vi "PIO.Read (U64).vi"(8 "error in (no error)":errorcluster, 10 "offset":u32 format="%.0x", 11 "GE 5565PIORC in":refnum<class "GE 5565PIORC.lvclass">) -> (0 "error out":errorcluster, 2 "value":u64, 3 "GE 5565PIORC out":refnum<class "GE 5565PIORC.lvclass">)   [LabVIEW 2016, in "GE 5565PIORC.lvclass"]
uses:
  GE 5565PIORC.lvclass
  GE 5565PIORC.lvclass/GE 5565PIORC.ctl
  <vilib>/Instr/_visa.llb/VISA Register Access Address Space.ctl
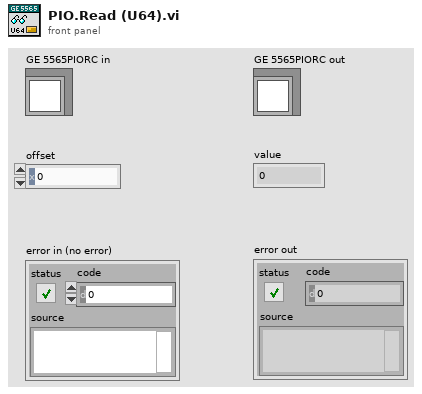
[diagram p1: front panel]
types:
  T1 = typedef "VISA Register Access Address Space.ctl" = u16
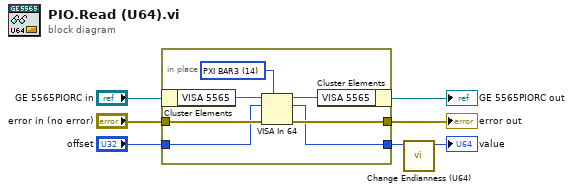
[diagram p0: block diagram]
diagram:
  n1 = in-place {
    in-place-border: "error in (no error)" -> [w14]
    in-place-border: [w13] -> w6
    in-place-border: "offset" -> [w9]
    in-place-border: [w8] -> w2
    w10 = T1 14 items=["VXI/VME A16"=1, "VXI/VME A24"=2, "VXI/VME A32"=3, "VXI/VME A64"=4, "PXI Memory Allocations"=9, "PXI Configuration"=10, "PXI BAR0"=11, "PXI BAR1"=12, "PXI BAR2"=13, "PXI BAR3"=14, "PXI BAR4"=15, "PXI BAR5"=16] ("Address Space")
    n2 = in-place-cluster #1("GE 5565PIORC in") -> ("VISA 5565"=w12:refnum<visa-resource-name>)
    n3 = VISA In 64(7:w10, 8:w14, 10:w9, 11:w12) -> (0:w13:errorcluster, 2:w8:u64, 3:w11:refnum<visa-resource-name>)
    n4 = in-place-cluster #1("VISA 5565"=w11) -> (→"GE 5565PIORC out":refnum<class "GE 5565PIORC.lvclass">)
  }
  "error out" <- w6
  n5 = call "Change Endianness (U64).vi"("number in"=w2) -> ("byte-reversed number out"=→"value":u64)  [unwired: 10 in]
